vi "OnFlatGround.vi"() -> (2 "OnFlatGround?":bool)   [LabVIEW 2015]
uses:
  navx-mxp/labview/navX Library v2/navX Library v2.lvlib
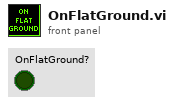
[diagram p1: front panel]
types:
  T1 = typedef "navX Library v2.lvlib/Z900_navX_DeviceTypeDef.ctl" = cluster{"Interface":cluster{"Protocol":T2, "Update Rate (4Hz-100Hz)":u8, "navX Open TypeDef":variant}, "Notify Packet":refnum<notifier>, "Loop VI Refnum":refnum<vi>, "Ready to Close Occurrence Refnum":refnum<k4>}
  T2 = typedef "navX Library v2.lvlib/Z900_navX_ProtocolTypeDef.ctl" = enum16{"SERIAL", "I2C", "SPI"}
  T3 = cluster{"Yaw":dbl, "Roll":dbl, "Pitch":dbl, "Heading":dbl, "Fused Heading":dbl}
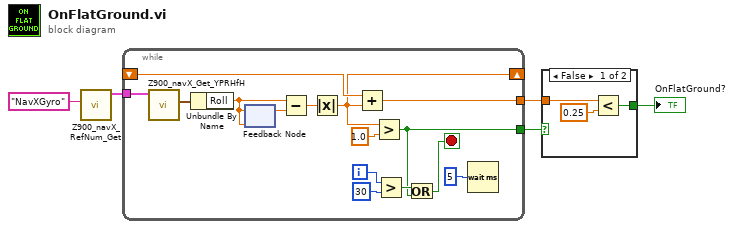
[diagram p0: block diagram]
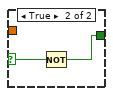
[diagram p2: hidden frame]
diagram:
  n1 = call "Z900_navX_RefNum_Get.vi"("refnum name"="NavXGyro") -> ("navX Device"=w4:T1)  [unwired: 9 in, 1 out]
  n2 = while {
    tunnel: w4 -> [w20]
    shift-right: [w8] -> _
    shift-left: _ -> [w18]
    tunnel: [w16] -> w3
    tunnel: [w6] -> w1
    i -> [w11]
    stop <- w9 stop-if-true
    n3 = call "Z900_navX_Get_YPRHfH.vi"("navX Device"=w20) -> ("YRPHfH"=w19:T3)  [unwired: 7 in, 3 out]
    n4 = Unbundle By Name(w19) -> ("Roll"=w14:dbl)
    n5 = feedback-in #1(w14) -> ()
    n6 = feedback #1(w14) -> (w15:dbl)
    n7 = Subtract(x=w14, y=w15) -> (x-y=w17:dbl)
    n8 = Absolute Value(x=w17) -> (abs(x)=w8:dbl)
    n9 = Add(x=w18, y=w8) -> (x+y=w16:dbl)
    n10 = Greater?(x=w8, y=1.0) -> (0:w6:bool)
    n11 = Greater?(x=w11, y=30) -> (0:w12:bool)
    n12 = Or(x=w12, y=w6) -> (x .or. y?=w9:bool)
    n13 = Wait (ms)(milliseconds to wait=u32 5) -> ()  [unwired: 1 out]
  }
  n14 = case shown="False" w1 {
    selector: w1 -> [_ w25]
    tunnel: w3 -> [w23 _]
    tunnel: [w21 w24] -> w2
    frame False {
      n15 = Less?(x=w23, y=0.25) -> (x < y?=w21:bool)
    }
    frame True {
      n16 = Not(x=w25) -> (.not. x?=w24:bool)
    }
  }
  "OnFlatGround?" <- w2
